vi "Set Radio Button (Value Sgnl).vi"(0 "Radio Buttons Ref In":refnum<vi>, 5 "Radio Button Text":string, 11 "error in (no error)":errorcluster) -> (6 "Found?":bool, 15 "error out":errorcluster)   [LabVIEW 2019]
doc: "Set Radio Buttons by Value Sgnl."
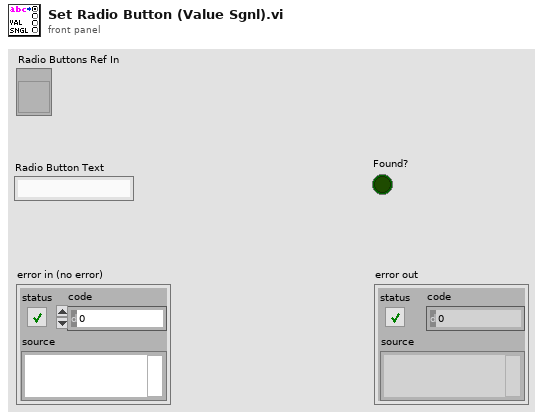
[diagram p1: front panel]
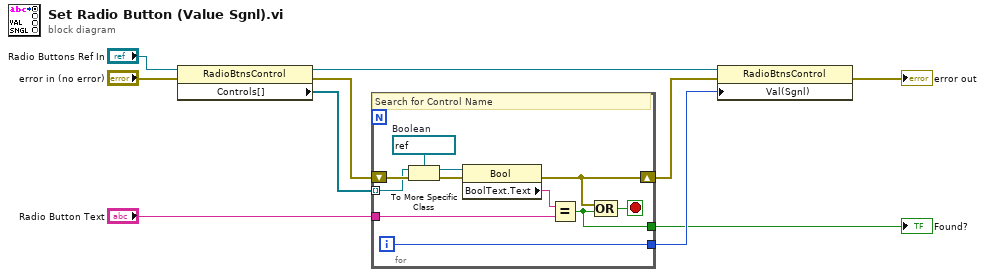
[diagram p0: block diagram]
diagram:
  n1 = property class="RadioBtnsControl"(reference="Radio Buttons Ref In", error in="error in (no error)") -> (reference out=w6:refnum<vi>, error out=w10:errorcluster, "Controls[]"=w9:refnum<vi>[])
  n2 = for {
    tunnel: w9 -> [w17] mode=indexing
    shift-right: [w15] -> w7
    shift-left: w10 -> [w18]
    tunnel: "Radio Button Text" -> [w13]
    tunnel: [w12] -> w5
    tunnel: [w11] -> w1
    i -> [w12]
    stop <- w14 stop-if-true
    w20 = refnum<vi> refnum  # Boolean
    # "Search for Control Name"
    n3 = To More Specific Class(target class=w20, reference=w17, error in=w18) -> (specific class reference=w19:refnum<vi>, error out=w21:errorcluster)
    n4 = property class="Bool"(reference=w19, error in=w21) -> (error out=w15:errorcluster, "BoolText.Text"=w16:string)  [unwired: 1 out]
    n5 = Equal?(x=w16, y=w13) -> (x = y?=w11:bool)
    n6 = Compound Arithmetic op=OR(w15, w11) -> (w14:bool)
  }
  "Found?" <- w1
  n7 = property class="RadioBtnsControl"(reference=w6, error in=w7, "Val(Sgnl)"=w5) -> (error out=→"error out":errorcluster)  [unwired: 1 out]
